vi "Read NMEA Compass SubVI.vi"(0 "VISA resource name":refnum<visa-resource-name>="COM1", 5 "timeout (ms)":u32=10000, 9 "stop":bool, 11 "error in (no error)":errorcluster) -> (4 "Heading":dbl, 10 "Stopped?":bool, 15 "error out":errorcluster)   [LabVIEW 2014]
doc: "This subVI decodes the most common NMEA-0183 sentence transmitted by GPS receivers, the $GPRMC sentence. The subvi returns time, position, ground speed, and magnetic variation. In the GPS interface configuration, use the \"NMEA OUT\" setting and set the baud rate to the standard 4800 bps setting. Connected to the computer's serial port using a PC Interface Cable, available from the GPS vendor. This subvi initializes the serial port on first call. On subsequent calls, the initialization is skipped. Always use the Stop input when stopping the VI so that the serial port connection is closed."
uses:
  <vilib>/Instr/_visa.llb/VISA Configure Serial Port (Instr).vi
panel:
  out "token output":string
  out "Data":string
  in  "stop the while":bool
  out "Bytes read":u32
  out "String Read":string="\n"
  # "I changed this to read compass:"
  # "This subVI decodes the most common NMEA-0183 sentence transmitted by GPS receivers, the $GPRMC sentence. The subvi returns time, position, ground speed, and magnetic variation. In the GPS interface configuration, use the \"NMEA OUT\" setting and set the baud rate to the standard 4800 bps setting. Connected to the computer's serial port using a PC Interface Cable, available from the GPS vendor. This subvi initializes the serial port on first call. On subsequent calls, the initialization is skipped. Always use the Stop input when stopping the VI so that the serial port connection is closed."
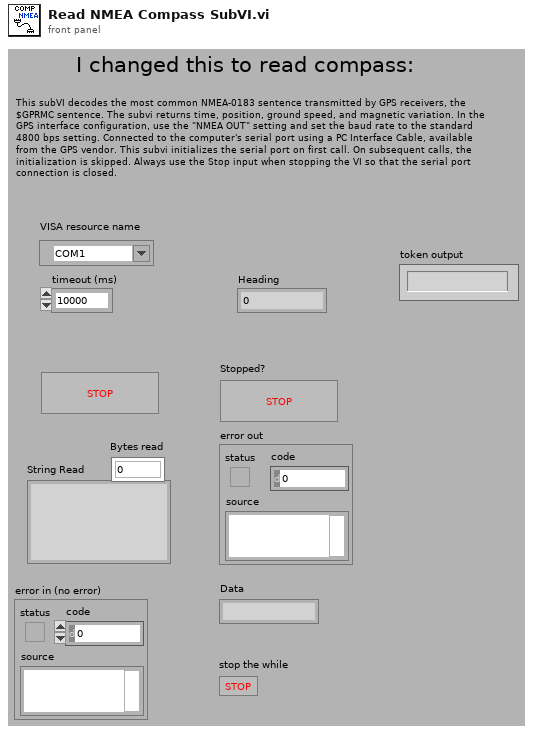
[diagram p1: front panel]
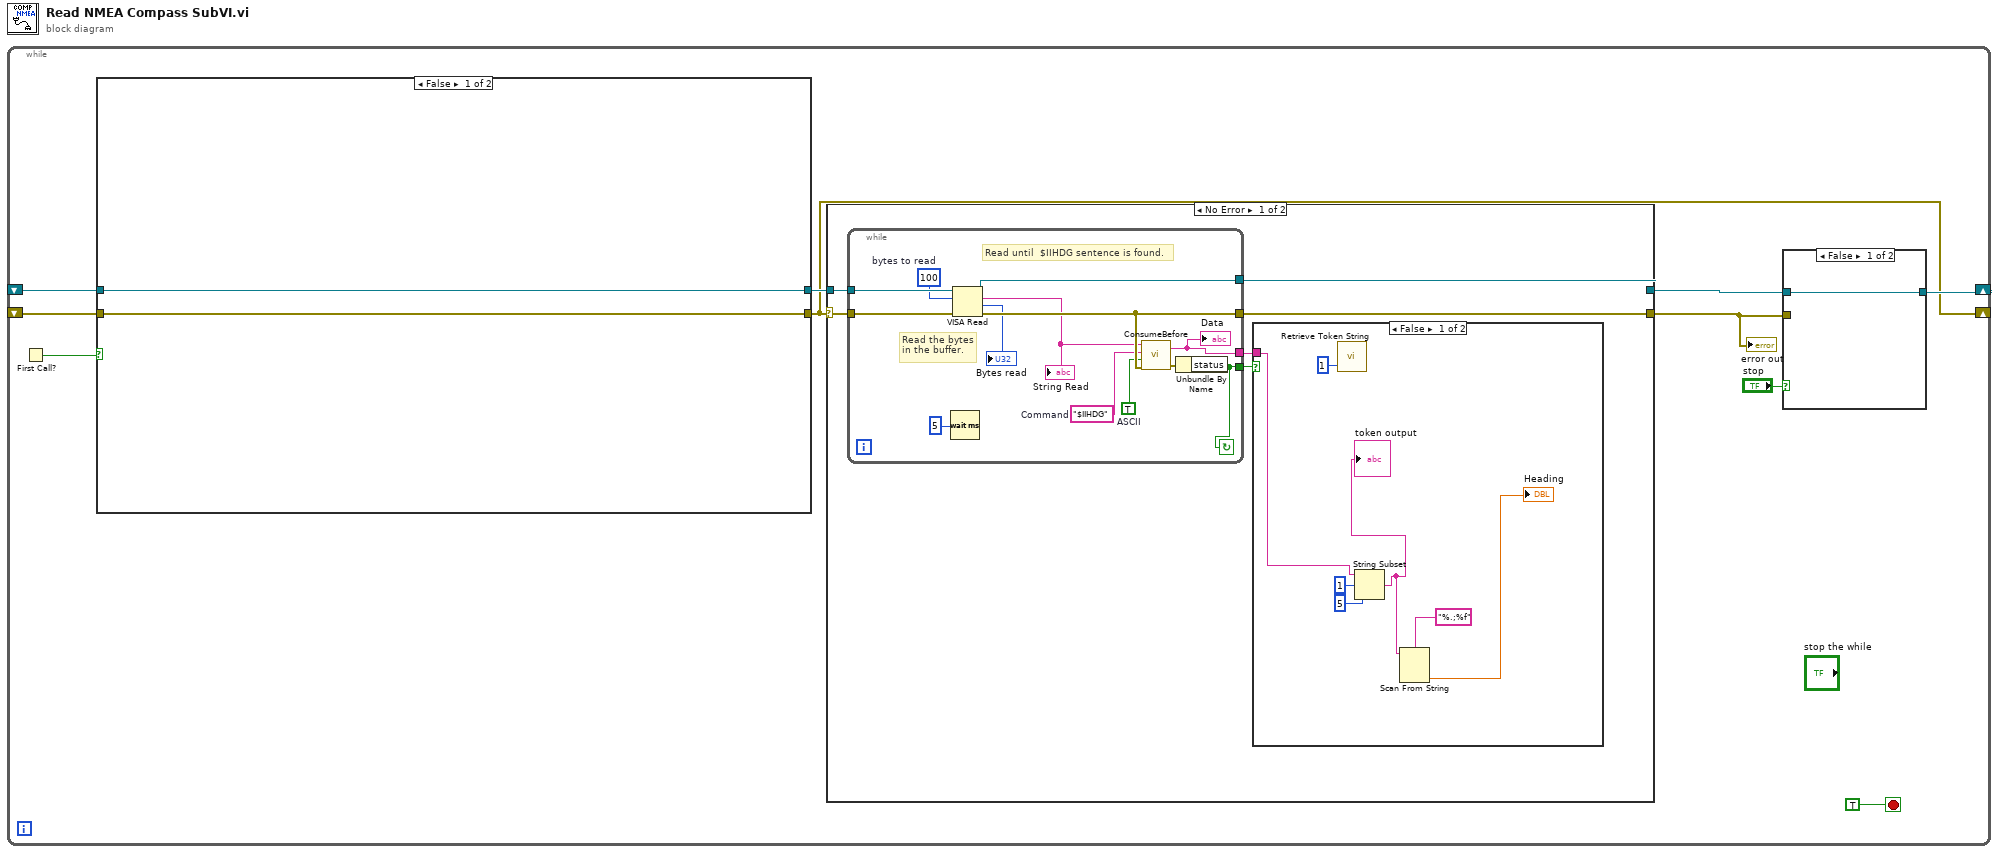
[diagram p0: block diagram]
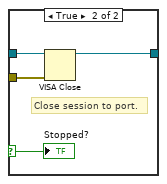
[diagram p2: hidden frame]
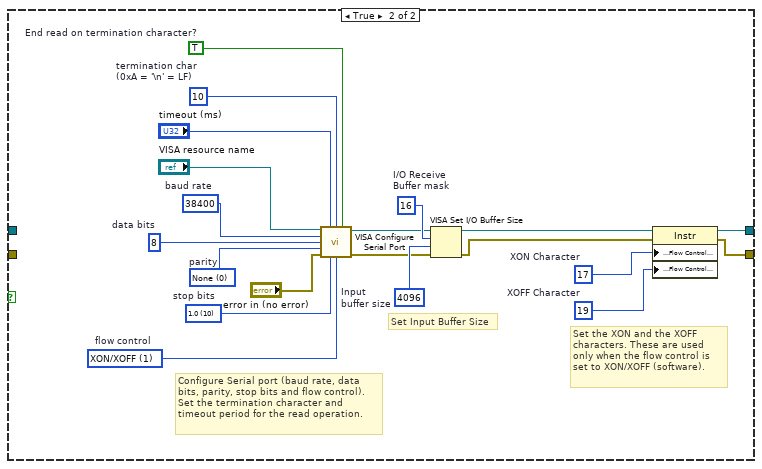
[diagram p3: hidden frame]
diagram:
  n1 = while {
    shift-right: [w6] -> _
    shift-left: _ -> [w5]
    shift-right: [w4] -> _
    shift-left: _ -> [w3]
    stop <- TRUE stop-if-true
    n2 = First Call?() -> (First Call?: T/F=w8:bool)
    n3 = case shown="False" w8 {
      tunnel: [w16 w21] -> w10
      tunnel: [w15 w18] -> w4
      tunnel: w5 -> [w16 _]
      tunnel: w3 -> [w15 _]
      frame False {
      }
      frame True {
        w31 = TRUE  # End read on termination character?
        w23 = u8 19  # XOFF Character
        w24 = u8 17  # XON Character
        w29 = u32 4096  # Input buffer size
        w27 = u16 1 items=["None"=0, "XON/XOFF"=1, "RTS/CTS"=2, "DTR/DSR"=4]  # flow control
        w33 = u16 10 items=["1.0"=10, "1.5"=15, "2.0"=20]  # stop bits
        w34 = u16 0 items=["None", "Odd", "Even", "Mark", "Space"]  # parity
        w22 = u16 8  # data bits
        w36 = u32 38400  # baud rate
        w28 = u8 10  # termination char (0xA = '\n' = LF)
        w30 = u16 16  # I/O Receive Buffer mask
        # "Set the XON and the XOFF\ncharacters. These are used\nonly when the flow control is\nset to XON/XOFF (software)."
        # "Configure Serial port (baud rate, data\nbits, parity, stop bits and flow control).\nSet the termination character and\ntimeout period for the read operation."
        # "Set Input Buffer Size"
        n4 = call-poly "VISA Configure Serial Port"("VISA resource name"="VISA resource name", "timeout (10sec)"="timeout (ms)", "termination char\n(0xA = '\\n' = LF)"=w28, "Enable Termination\nChar (T)"=w31, "baud rate (9600)"=w36, "data bits (8)"=w22, "parity (0:none)"=w34, "error in (no error)"="error in (no error)", "stop bits (10: 1 bit)"=w33, "flow control (0:none)"=w27) -> ("VISA resource name out"=w20:refnum<visa-resource-name>, "error out"=w19:errorcluster)  [unwired: 4 in]
        n5 = VISA Set I/O Buffer Size(VISA resource name=w20, mask (16)=w30, size (4096)=w29, error in (no error)=w19) -> (VISA resource name out=w26:refnum<visa-resource-name>, error out=w25:errorcluster)
        n6 = property class="Instr"(reference=w26, error in=w25, "Serial Settings:Flow Control XON Character"=w24, "Serial Settings:Flow Control XOFF Character"=w23) -> (reference out=w21:refnum<visa-resource-name>, error out=w18:errorcluster)
      }
    }
    n7 = case shown="No Error" w4 {
      selector: w4 -> [w39 w63]
      tunnel: w10 -> [w42 w64]
      tunnel: [w41 w64] -> w9
      tunnel: [w40 w63] -> w2
      frame No Error {
        n8 = while {
          tunnel: w42 -> [w55]
          tunnel: [w54] -> w41
          tunnel: [w53] -> w40
          tunnel: w39 -> [w52]
          tunnel: [w43] -> w38
          tunnel: [w44] -> w37
          stop <- w44 continue-if-true
          w47 = u32 100  # bytes to read
          w51 = "$IIHDG"  # Command
          w50 = TRUE  # ASCII
          # "Read until  $IIHDG sentence is found."
          # "Read the bytes\nin the buffer."
          n9 = Wait (ms)(milliseconds to wait=u32 5 ("millisecond multiple")) -> ()  [unwired: 1 out]
          n10 = VISA Read(VISA resource name=w55, byte count=w47, error in (no error)=w52) -> (VISA resource name out=w54:refnum<visa-resource-name>, read buffer=w49:string, return count=→"Bytes read":u32, error out=w53:errorcluster)
          "String Read" <- w49
          n11 = call "ConsumeBefore.vi"("error in"=w53, "ASCII"=w50, "Before"=w51, "Response String In"=w49) -> ("error out"=w48:errorcluster, "Response String Out"=w43:string)
          "Data" <- w43
          n12 = Unbundle By Name(w48) -> ("status"=w44:bool)
        }
        n13 = case shown="False" w37 {
          tunnel: w38 -> [w59 _]
          frame False {
            n14 = call "Retrieve Token String.vi"("Offset (0)"=1) -> ()  [unwired: 1 in, 2 out]
            n15 = String Subset(string=w59, offset (0)=1, length (rest)=5 ("length (rest)")) -> (substring=w56:string)
            "token output" <- w56
            n16 = Scan From String(format string="%.;%f", input string=w56) -> (output 1=→"Heading":dbl)  [unwired: 3 in, 3 out]
          }
          frame True {
          }
        }
      }
      frame Error {
      }
    }
    "error out" <- w2
    n17 = case shown="False" "stop" {
      selector: "stop" -> [_ w12]
      tunnel: w9 -> [w11 w13]
      tunnel: w2 -> [_ w14]
      tunnel: [w11 w13] -> w6
      frame False {
      }
      frame True {
        # "Close session to port."
        n18 = VISA Close(VISA resource name=w13, error in (no error)=w14) -> ()  [unwired: 1 out]
        "Stopped?" <- w12
      }
    }
  }
